vi "TestM1M3SALTelemetryTiming.vi"() -> ()   [LabVIEW 2016]
uses:
  Communicator/M1M3SAL/M1M3SAL.lvclass
  Communicator/DataTypes/M1M3SALSettings.ctl
  UserEvents/UserEvents.lvclass
  DataTypes/Topics/TelemetryFPGAData.ctl
  DataTypes/Topics/Parts/Timestamp.ctl
  Communicator/M1M3SAL/M1M3SAL.lvclass/M1M3SAL.ctl
  Communicator/M1M3SupportCommunicator.lvlib
  DataTypes/Topics/M1M3SupportTopics.lvlib
panel:
  out "Iteration":i32
  out "Time":u32
  in  "Boolean":bool
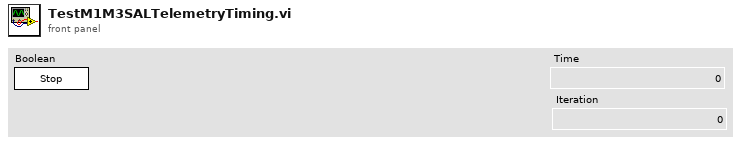
[diagram p1: front panel]
types:
  T1 = typedef "M1M3SupportCommunicator.lvlib/M1M3SALSettings.ctl" = cluster{"IPAddress":string, "Port":u16, "StartupScript":string}
  T2 = typedef "M1M3SupportTopics.lvlib/TelemetryFPGAData.ctl" = cluster{"Timestamp":T3, "ModbusSubnetATxInternalFIFOOverflow":bool, "ModbusSubnetAInvalidInstruction":bool, "ModbusSubnetAWaitForRxFrameTimeout":bool, "ModbusSubnetAStartBitError":bool, "ModbusSubnetAStopBitError":bool, "ModbusSubnetARxDataFIFOOverflow":bool, "ModbusSubnetATxByteCount":u32, "ModbusSubnetATxFrameCount":u32, "ModbusSubnetARxByteCount":u32, "ModbusSubnetARxFrameCount":u32, "ModbusSubnetBTxInternalFIFOOverflow":bool, "ModbusSubnetBInvalidInstruction":bool, "ModbusSubnetBWaitForRxFrameTimeout":bool, "ModbusSubnetBStartBitError":bool, "ModbusSubnetBStopBitError":bool, "ModbusSubnetBRxDataFIFOOverflow":bool, "ModbusSubnetBTxByteCount":u32, "ModbusSubnetBTxFrameCount":u32, "ModbusSubnetBRxByteCount":u32, "ModbusSubnetBRxFrameCount":u32, "ModbusSubnetCTxInternalFIFOOverflow":bool, "ModbusSubnetCInvalidInstruction":bool, "ModbusSubnetCWaitForRxFrameTimeout":bool, "ModbusSubnetCStartBitError":bool, "ModbusSubnetCStopBitError":bool, "ModbusSubnetCRxDataFIFOOverflow":bool, "ModbusSubnetCTxByteCount":u32, "ModbusSubnetCTxFrameCount":u32, "ModbusSubnetCRxByteCount":u32, "ModbusSubnetCRxFrameCount":u32, "ModbusSubnetDTxInternalFIFOOverflow":bool, "ModbusSubnetDInvalidInstruction":bool, "ModbusSubnetDWaitForRxFrameTimeout":bool, "ModbusSubnetDStartBitError":bool, "ModbusSubnetDStopBitError":bool, "ModbusSubnetDRxDataFIFOOverflow":bool, "ModbusSubnetDTxByteCount":u32, "ModbusSubnetDTxFrameCount":u32, "ModbusSubnetDRxByteCount":u32, "ModbusSubnetDRxFrameCount":u32, "ModbusSubnetETxInternalFIFOOverflow":bool, "ModbusSubnetEInvalidInstruction":bool, "ModbusSubnetEWaitForRxFrameTimeout":bool, "ModbusSubnetEStartBitError":bool, "ModbusSubnetEStopBitError":bool, "ModbusSubnetERxDataFIFOOverflow":bool, "ModbusSubnetETxByteCount":u32, "ModbusSubnetETxFrameCount":u32, "ModbusSubnetERxByteCount":u32, "ModbusSubnetERxFrameCount":u32, "FPGATimestamp":dbl}
  T3 = typedef "M1M3SupportTopics.lvlib/Timestamp.ctl" = dbl
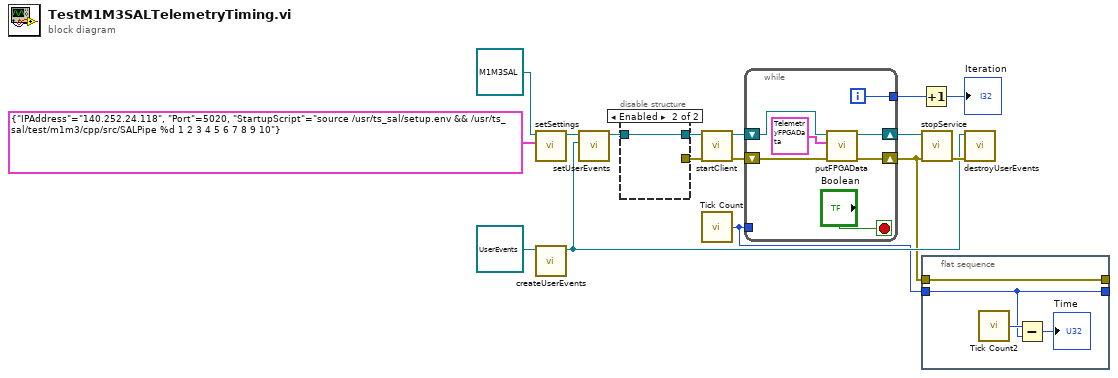
[diagram p0: block diagram]
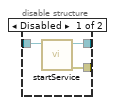
[diagram p2: hidden frame]
diagram:
  n1 = call "setSettings.vi"("Settings"=T1 {"IPAddress"="140.252.24.118", "Port"=5020, "StartupScript"="source /usr/ts_sal/setup.env && /usr/ts_sal/test/m1m3/cpp/src/SALPipe %d 1 2 3 4 5 6 7 8 9 10"}, "M1M3SAL in"=refnum<class "M1M3SAL.lvclass"> refnum ("M1M3SupportCommunicator.lvlib:M1M3SAL.lvclass")) -> ("M1M3SAL out"=w13:refnum<class "M1M3SAL.lvclass">)  [unwired: 9 in]
  n2 = call "createUserEvents.vi"("UserEvents in"=refnum<class "UserEvents.lvclass"> refnum ("UserEvents.lvclass")) -> ("UserEvents out"=w6:refnum<class "UserEvents.lvclass">)  [unwired: 9 in, 1 out]
  n3 = call "setUserEvents.vi"("UserEvents"=w6, "M1M3SAL in"=w13) -> ("M1M3SAL out"=w12:refnum<class "M1M3SAL.lvclass">)  [unwired: 9 in]
  n4 = disable-structure shown="Enabled" {
    disable-tunnel: w12 -> [w19 w20]
    disable-tunnel: [w18 w20] -> w11
    disable-tunnel: [w17 _] -> w10
    frame Disabled {
      n5 = call-dynamic "startService.vi"("M1M3SAL in"=w19) -> ("error out"=w17:errorcluster, "M1M3SAL out"=w18:refnum<class "M1M3SAL.lvclass">)  [unwired: 9 in]
    }
    frame Enabled {
    }
  }
  n6 = call-dynamic "startClient.vi"("error in (no error)"=w10, "M1M3SAL in"=w11) -> ("error out"=w5:errorcluster, "M1M3SAL out"=w9:refnum<class "M1M3SAL.lvclass">)  [unwired: 8 in]
  n7 = call "Tick Count"() -> ("Tick Count(uSec)"=w1:u32)
  n8 = while {
    shift-right: [w26] -> w8
    shift-left: w9 -> [w27]
    shift-right: [w25] -> w2
    shift-left: w5 -> [w22]
    tunnel: w1 -> [_]
    tunnel: [w21] -> w3
    i -> [w21]
    stop <- "Boolean" stop-if-true
    n9 = call-dynamic "putFPGAData.vi"("error in (no error)"=w22, "TelemetryFPGAData"=T2 {"Timestamp"=1.0, "ModbusSubnetATxInternalFIFOOverflow"=TRUE, "ModbusSubnetAInvalidInstruction"=FALSE, "ModbusSubnetAWaitForRxFrameTimeout"=TRUE, "ModbusSubnetAStartBitError"=FALSE, "ModbusSubnetAStopBitError"=TRUE, "ModbusSubnetARxDataFIFOOverflow"=FALSE, "ModbusSubnetATxByteCount"=8, "ModbusSubnetATxFrameCount"=9, "ModbusSubnetARxByteCount"=10, "ModbusSubnetARxFrameCount"=11, "ModbusSubnetBTxInternalFIFOOverflow"=TRUE, "ModbusSubnetBInvalidInstruction"=FALSE, "ModbusSubnetBWaitForRxFrameTimeout"=TRUE, "ModbusSubnetBStartBitError"=FALSE, "ModbusSubnetBStopBitError"=TRUE, "ModbusSubnetBRxDataFIFOOverflow"=FALSE, "ModbusSubnetBTxByteCount"=18, "ModbusSubnetBTxFrameCount"=19, "ModbusSubnetBRxByteCount"=20, "ModbusSubnetBRxFrameCount"=21, "ModbusSubnetCTxInternalFIFOOverflow"=TRUE, "ModbusSubnetCInvalidInstruction"=FALSE, "ModbusSubnetCWaitForRxFrameTimeout"=TRUE, "ModbusSubnetCStartBitError"=FALSE, "ModbusSubnetCStopBitError"=TRUE, "ModbusSubnetCRxDataFIFOOverflow"=FALSE, "ModbusSubnetCTxByteCount"=28, "ModbusSubnetCTxFrameCount"=29, "ModbusSubnetCRxByteCount"=30, "ModbusSubnetCRxFrameCount"=31, "ModbusSubnetDTxInternalFIFOOverflow"=TRUE, "ModbusSubnetDInvalidInstruction"=FALSE, "ModbusSubnetDWaitForRxFrameTimeout"=TRUE, "ModbusSubnetDStartBitError"=FALSE, "ModbusSubnetDStopBitError"=TRUE, "ModbusSubnetDRxDataFIFOOverflow"=FALSE, "ModbusSubnetDTxByteCount"=38, "ModbusSubnetDTxFrameCount"=39, "ModbusSubnetDRxByteCount"=40, "ModbusSubnetDRxFrameCount"=41, "ModbusSubnetETxInternalFIFOOverflow"=TRUE, "ModbusSubnetEInvalidInstruction"=FALSE, "ModbusSubnetEWaitForRxFrameTimeout"=TRUE, "ModbusSubnetEStartBitError"=FALSE, "ModbusSubnetEStopBitError"=TRUE, "ModbusSubnetERxDataFIFOOverflow"=FALSE, "ModbusSubnetETxByteCount"=48, "ModbusSubnetETxFrameCount"=49, "ModbusSubnetERxByteCount"=50, "ModbusSubnetERxFrameCount"=51, "FPGATimestamp"=52.0}, "M1M3SAL in"=w27) -> ("error out"=w25:errorcluster, "M1M3SAL out"=w26:refnum<class "M1M3SAL.lvclass">)  [unwired: 7 in]
  }
  n10 = Increment(x=w3) -> (x+1=→"Iteration":i32)
  n11 = call-dynamic "stopService.vi"("error in (no error)"=w2, "M1M3SAL in"=w8) -> ("error out"=w7:errorcluster)  [unwired: 8 in, 1 out]
  n12 = flat-sequence {
    tunnel: [w31] -> _
    tunnel: w2 -> [w31]
    tunnel: [w28] -> _
    tunnel: w1 -> [w28]
    frame #0 {
      n13 = call "Tick Count2"() -> ("Tick Count(uSec)"=w30:u32)
      n14 = Subtract(x=w30, y=w28) -> (x-y=→"Time":u32)
    }
  }
  n15 = call "destroyUserEvents.vi"("error in (no error)"=w7, "UserEvents in"=w6) -> ()  [unwired: 8 in, 2 out]
